vi "Finish Autofocus.vi"(8 "error in (no error)":errorcluster, 11 "Application in":refnum<class "Application.lvclass">) -> (0 "error out":errorcluster, 3 "Application out":refnum<class "Application.lvclass">)   [LabVIEW 2018, in "Application.lvlib" / "Application.lvclass"]
uses:
  Application.lvclass
  <vilib>/Analysis/NI_AALPro.lvlib
panel:
  out "Brenner Gradient":dbl[](array[numeric])
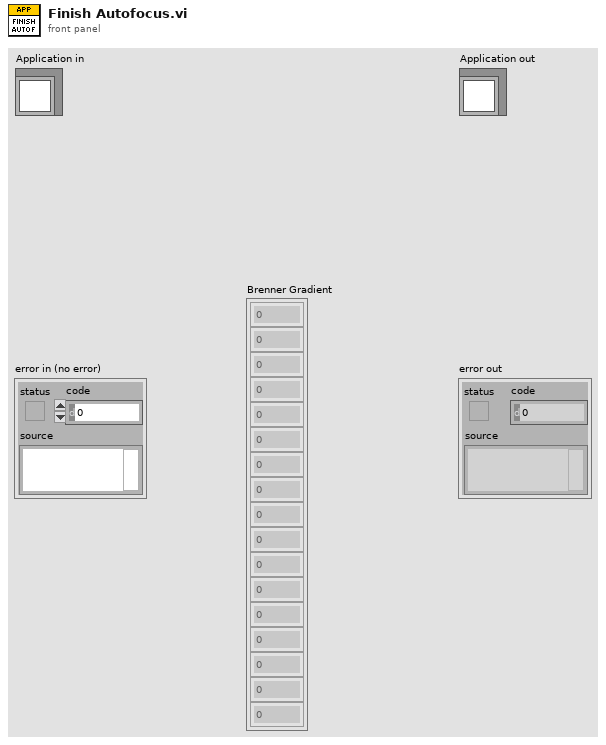
[diagram p1: front panel]
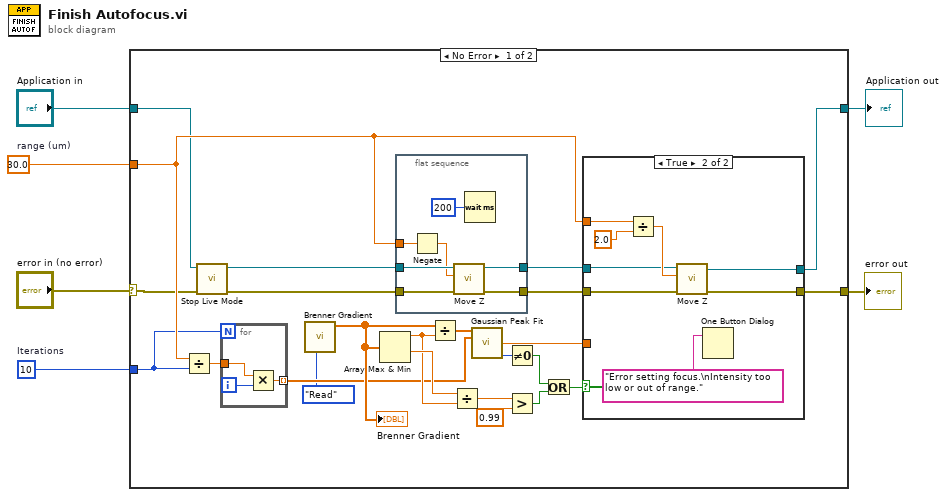
[diagram p0: block diagram]
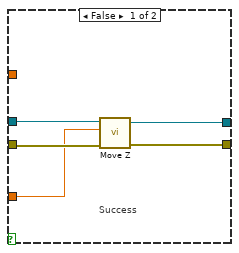
[diagram p2: hidden frame]
diagram:
  w2 = 30.0  # range (um)
  w1 = 10  # Iterations
  n1 = case shown="No Error" "error in (no error)" {
    selector: "error in (no error)" -> [w13 w55]
    tunnel: [w9 w55] -> w5
    tunnel: [w8 w54] -> w3
    tunnel: "Application in" -> [w12 w54]
    tunnel: w2 -> [w17 _]
    tunnel: w1 -> [w16 _]
    frame No Error {
      n2 = Divide(x=w17, y=w16) -> (x/y=w15:dbl)
      n3 = call-dynamic "Stop Live Mode.vi"("error in (no error)"=w13, "Application in"=w12) -> ("error out"=w10:errorcluster, "Application out"=w11:refnum<class "Application.lvclass">)  [unwired: 8 in]
      n4 = for {
        N: w16 -> [_]
        tunnel: w15 -> [w40]
        tunnel: [w38] -> w14 mode=indexing
        i -> [w39]
        n5 = Multiply(x=w40, y=w39) -> (x*y=w38:dbl)
      }
      n6 = call "Brenner Gradient.vi"("Enum"=enum16{"Reset", "Read", "Write"}."Read") -> ("Brenner Gradients"=w18:dbl[])  [unwired: 10 in]
      "Brenner Gradient" <- w18
      n7 = Array Max & Min(array=w18) -> (max value=w28:dbl, min value=w29:dbl)  [unwired: 2 out]
      n8 = flat-sequence "Move down first to ensure motor is engaged" {
        tunnel: w10 -> [w34]
        tunnel: w11 -> [w36]
        tunnel: w17 -> [w37]
        tunnel: [w32] -> w19
        tunnel: [w33] -> w21
        frame #0 {
          n9 = Negate(x=w37) -> (-x=w35:dbl)
          n10 = call-dynamic "Move Z.vi"("error in (no error)"=w34, "Delta (um)"=w35, "Application in"=w36) -> ("error out"=w33:errorcluster, "Application out"=w32:refnum<class "Application.lvclass">)  [unwired: 7 in]
          n11 = Wait (ms)(milliseconds to wait=u32 200) -> ()  [unwired: 1 out]
        }
      }
      n12 = Divide(x=w18, y=w28) -> (x/y=w26:dbl[])
      n13 = Divide(x=w29, y=w28) -> (x/y=w30:dbl)
      n14 = call <vilib>:"Gaussian Peak Fit.vi"("Y"=w26, "X"=w14) -> ("center"=w20:dbl, "error"=w24:i32)  [unwired: 7 in, 5 out]
      n15 = Not Equal To 0?(x=w24) -> (x != 0?=w23:bool)
      n16 = Greater?(x=w30, y=0.99) -> (0:w25:bool)
      n17 = Or(x=w23, y=w25) -> (x .or. y?=w22:bool)
      n18 = case shown="True" w22 {
        tunnel: w21 -> [w43 w49]
        tunnel: w20 -> [w41 _]
        tunnel: w19 -> [w44 w47]
        tunnel: [w42 w50] -> w9
        tunnel: w17 -> [_ w53]
        tunnel: [w45 w46] -> w8
        frame False {
          # "Success"
          n19 = call-dynamic "Move Z.vi"("error in (no error)"=w43, "Delta (um)"=w41, "Application in"=w44) -> ("error out"=w42:errorcluster, "Application out"=w45:refnum<class "Application.lvclass">)  [unwired: 7 in]
        }
        frame True {
          n20 = Divide(x=w53, y=2.0) -> (x/y=w48:dbl)
          n21 = call-dynamic "Move Z.vi"("error in (no error)"=w49, "Delta (um)"=w48, "Application in"=w47) -> ("error out"=w50:errorcluster, "Application out"=w46:refnum<class "Application.lvclass">)  [unwired: 7 in]
          n22 = One Button Dialog(message="Error setting focus.\nIntensity too low or out of range.") -> ()  [unwired: 1 in, 1 out]
        }
      }
    }
    frame Error {
    }
  }
  "error out" <- w5
  "Application out" <- w3
